vi "Centre Position Values.vi"(0 "Position Values":cluster{dbl[], dbl[]}) -> (1 "Centred Position Values":cluster{dbl[], dbl[]}, 2 "Translation":cluster{"mean":dbl, "mean":dbl})   [LabVIEW 2013]
uses:
  <vilib>/Analysis/baseanly.llb/Mean (DBL).vi
  <vilib>/Analysis/NI_AALBase.lvlib
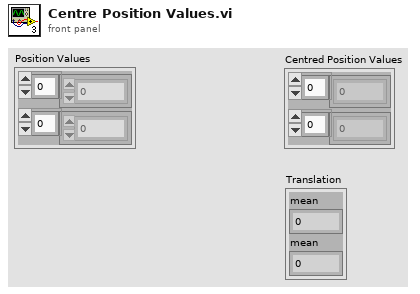
[diagram p1: front panel]
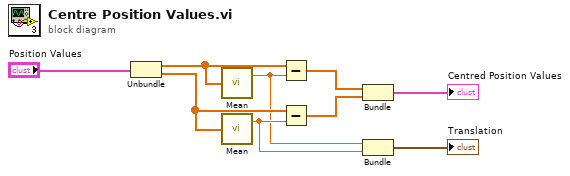
[diagram p0: block diagram]
diagram:
  n1 = Unbundle("Position Values") -> (w8:dbl[], w9:dbl[])
  n2 = call-poly <vilib>:"Mean.vi"("X"=w8) -> ("mean"=w5:dbl)  [unwired: 1 out]
  n3 = call-poly <vilib>:"Mean.vi"("X"=w9) -> ("mean"=w6:dbl)  [unwired: 1 out]
  n4 = Subtract(x=w8, y=w5) -> (x-y=w1:dbl[])
  n5 = Subtract(x=w9, y=w6) -> (x-y=w2:dbl[])
  n6 = Bundle(w1, w2) -> (→"Centred Position Values":cluster{dbl[], dbl[]})  [unwired: 1 in]
  n7 = Bundle("mean"=w5, "mean"=w6) -> (→"Translation":cluster{"mean":dbl, "mean":dbl})  [unwired: 1 in]
